vi "Open Actor Core FP.vi"(8 "error in (no error)":errorcluster, 10 "Open FP (F)":bool, 11 "CS++BaseActor in":refnum<class "CS++BaseActor.lvclass">) -> (0 "error out":errorcluster, 3 "CS++BaseActor out":refnum<class "CS++BaseActor.lvclass">)   [LabVIEW 2014, in "CS++BaseActor.lvlib" / "CS++BaseActor.lvclass"]
doc: "Open or close <b>Actor Core.vi</B> frontpanel."
uses:
  CS++BaseActor.lvclass
  CS++BaseActor.lvclass/CS++BaseActor.ctl
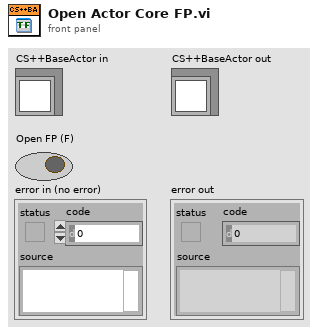
[diagram p1: front panel]
types:
  T1 = enum32{"Invalid", "Standard", "Closed", "Hidden", "Minimized", "Maximized"}
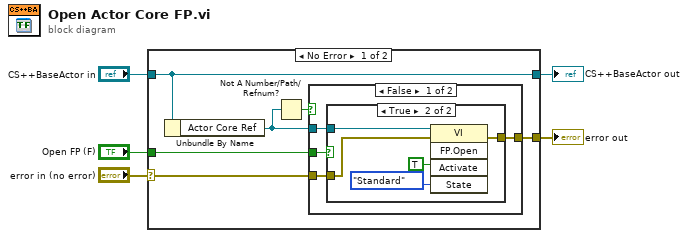
[diagram p0: block diagram]
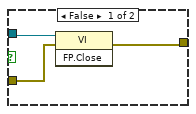
[diagram p2: hidden frame]
diagram:
  n1 = case shown="No Error" "error in (no error)" {
    selector: "error in (no error)" -> [w9 w26]
    tunnel: [w8 w26] -> w4
    tunnel: [w10 w25] -> w2
    tunnel: "CS++BaseActor in" -> [w10 w25]
    tunnel: "Open FP (F)" -> [w11 _]
    frame No Error {
      n2 = Unbundle By Name(w10) -> ("Actor Core Ref"=w6:refnum<vi>)
      n3 = Not A Number/Path/Refnum?(number/path/refnum=w6) -> (NaN/Path/Refnum?=w7:bool)
      n4 = case shown="False" w7 {
        tunnel: w11 -> [w15 _]
        tunnel: w6 -> [w14 _]
        tunnel: w9 -> [w13 w24]
        tunnel: [w12 w24] -> w8
        frame False {
          n5 = case shown="True" w15 {
            tunnel: w14 -> [w18 w21]
            tunnel: w13 -> [w17 w20]
            tunnel: [w16 w19] -> w12
            frame False {
              n6 = invoke class="VI" method="FP.Close"(reference=w18, error in=w17) -> (error out=w16:errorcluster)  [unwired: 1 in, 2 out]
            }
            frame True {
              n7 = invoke class="VI" method="FP.Open"(reference=w21, error in=w20, "Activate"=TRUE ("Activate?"), "State"=T1."Standard") -> (error out=w19:errorcluster)  [unwired: 1 in, 4 out]
            }
          }
        }
        frame True {
        }
      }
    }
    frame Error {
    }
  }
  "error out" <- w4
  "CS++BaseActor out" <- w2
